vi "fgPaths.vi"(7 "cmd":enum16{"init", "set", "get"}(ring), 8 "error in (no error)":errorcluster, 11 "clPaths":cluster{"Templates":path, "Reports":path}) -> (0 "error out":errorcluster, 3 "clPaths":cluster{"Templates":path, "Reports":path})   [LabVIEW 2014]
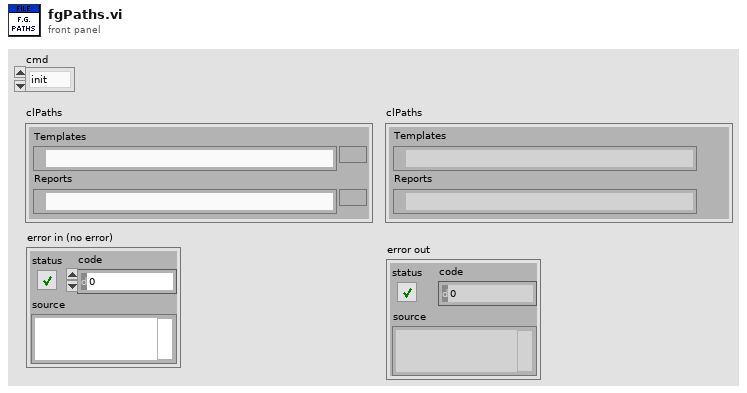
[diagram p1: front panel]
types:
  T1 = enum32{"invalid app kind", "Development System", "Run Time System", "Student Edition", "Embedded LabVIEW", "Evaluation", "Custom"}
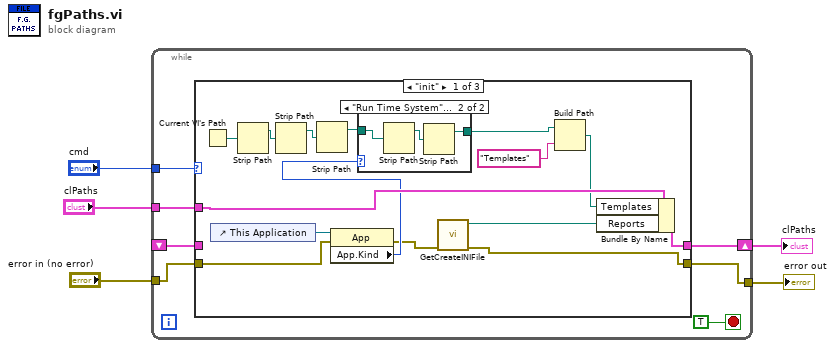
[diagram p0: block diagram]
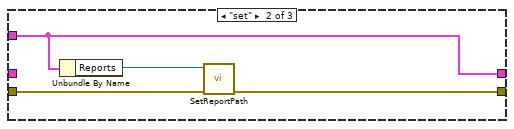
[diagram p3: hidden frame]
diagram:
  n1 = while {
    shift-right: [w9] -> w5
    shift-left: _ -> [w8]
    tunnel: "clPaths" -> [w10]
    tunnel: "cmd" -> [w11]
    tunnel: "error in (no error)" -> [w7]
    tunnel: [w6] -> w1
    stop <- TRUE stop-if-true
    n2 = case shown="\"init\"" w11 {
      tunnel: w10 -> [w24 w35 _]
      tunnel: [w22 w35 w37] -> w9
      tunnel: w8 -> [_ _ w37]
      tunnel: w7 -> [w21 w34 w36]
      tunnel: [w15 w33 w36] -> w6
      frame "init" {
        n3 = Current VI's Path() -> (path=w25:path)
        n4 = control-ref of="This Application"() -> (w20:refnum<vi>)
        n5 = Strip Path(path=w25) -> (stripped path=w27:path)  [unwired: 1 out]
        n6 = Strip Path(path=w27) -> (stripped path=w14:path)  [unwired: 1 out]
        n7 = Strip Path(path=w14) -> (stripped path=w13:path)  [unwired: 1 out]
        n8 = property class="App"(reference=w20, error in=w21) -> (error out=w17:errorcluster, "App.Kind"=w19:T1)  [unwired: 1 out]
        n9 = case shown="\"Run Time System\", Default" w19 {
          tunnel: w13 -> [w28 w29]
          tunnel: [w28 w31] -> w18
          frame "Development System" {
          }
          frame "Run Time System", Default {
            n10 = Strip Path(path=w29) -> (stripped path=w30:path)  [unwired: 1 out]
            n11 = Strip Path(path=w30) -> (stripped path=w31:path)  [unwired: 1 out]
          }
        }
        n12 = call "GetCreateINIFile.vi"("error in (no error)"=w17) -> ("error out"=w15:errorcluster, "ReportPath"=w16:path)  [unwired: 9 in]
        n13 = Build Path(base path=w18, name or relative path="Templates" ("string")) -> (appended path=w23:path)
        n14 = Bundle By Name(cluster=w24, "Templates"=w23, "Reports"=w16) -> (w22:cluster{"Templates":path, "Reports":path})
      }
      frame "set" {
        n15 = Unbundle By Name(w35) -> ("Reports"=w32:path)
        n16 = call "SetReportPath.vi"("error in (no error)"=w34, "default path"=w32) -> ("error out"=w33:errorcluster)  [unwired: 8 in, 1 out]
      }
      frame "get", Default {
      }
    }
  }
  "clPaths" <- w5
  "error out" <- w1
